vi "Prediction Interval (Log).vi"(0 "Y":dbl[](array[numeric]), 1 "confidence level":dbl=0.95 format="%.2f", 5 "X":dbl[](array[numeric]), 7 "Weight":dbl[](array[numeric]), 9 "amplitude":dbl, 11 "scale":dbl, 12 "base":dbl(ring)=2.71828 items=["e"=2.71828, "2"=2.0, "10"=10.0]) -> (4 "Upper Bound":dbl[](array[numeric]), 6 "Lower Bound":dbl[](array[numeric]), 15 "error":i32)   [LabVIEW 2020, in "NI_AALPro.lvlib"]
doc: "Calculates statistical intervals of the best logarithmic fit for a data set (<B>X</B>, <B>Y</B>). You must manually select the polymorphic instance to use."
uses:
  <vilib>/Analysis/NI_AALPro.lvlib
  <resource>/lvanlys.dll
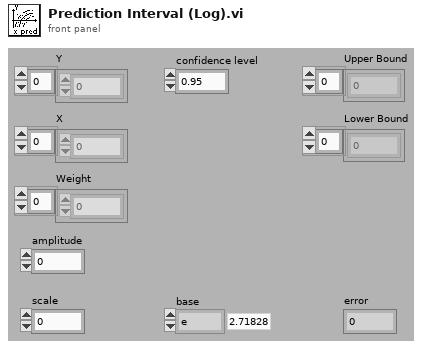
[diagram p1: front panel]
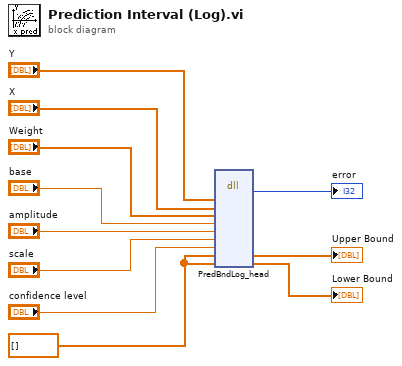
[diagram p0: block diagram]
diagram:
  w5 = dbl[] [] ("Best Linear Fit")
  n1 = dll-call lib="e:/builds/penguin/labview/branches/2020/dev/dist/resource/lvanlys.*" fn="PredBndLog_head"("y"="Y", "x"="X", "weight"="Weight", "base"="base", "amplitude"="amplitude", "scale"="scale", "confidentLevel"="confidence level", "upper"=w5, "lower"=w5) -> (→"error":i32, "upper"=→"Upper Bound":dbl[], "lower"=→"Lower Bound":dbl[])  [unwired: 10 in, 2 out]
